vi "mod_truncate phase noise.vi"(0 "phase noise in":cluster{"f0":dbl, "df":dbl, "magnitude":dbl[]} {"f0" format="%.2p"; "df" format="%.2p"; "magnitude" format="%.2p"}, 5 "offset stop (Hz)":dbl=1000000.0 format="%.2p", 11 "error in (no error)":errorcluster) -> (4 "phase noise out (truncated)":cluster{"f0":dbl, "df":dbl, "magnitude":dbl[]} {"f0" format="%.2p"; "df" format="%.2p"; "magnitude" format="%.2p"}, 15 "error out":errorcluster)   [LabVIEW 2020, in "niAMT.lvlib"]
uses:
  <vilib>/addons/Modulation/niAMT.lvlib
panel:
  in  "offset stop (Hz)":dbl=900000.0 format="%.2p"
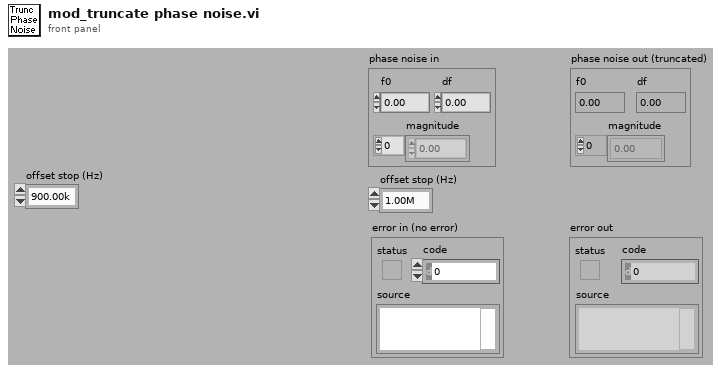
[diagram p1: front panel]
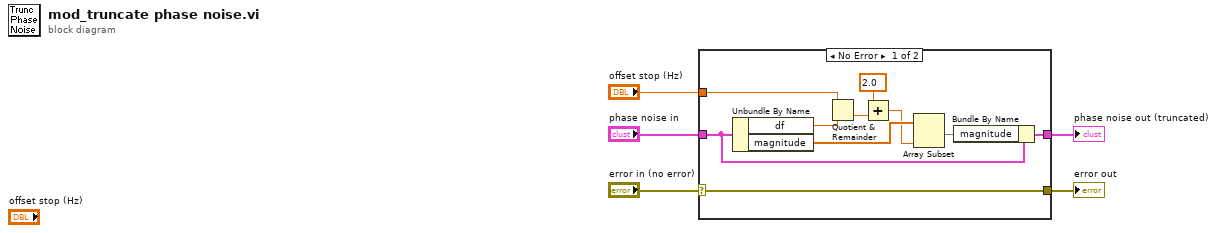
[diagram p0: block diagram]
diagram:
  n1 = case shown="No Error" "error in (no error)" {
    selector: "error in (no error)" -> [w6 w16]
    tunnel: "phase noise in" -> [w9 w17]
    tunnel: "offset stop (Hz)" -> [w8 _]
    tunnel: [w7 w17] -> w3
    tunnel: [w6 w16] -> w1
    frame No Error {
      n2 = Unbundle By Name(w9) -> ("df"=w15:dbl, "magnitude"=w14:dbl[])
      n3 = Quotient & Remainder(x=w8, y=w15) -> (floor(x/y)=w12:dbl)  [unwired: 1 out]
      n4 = Add(x=2.0, y=w12) -> (x+y=w10:dbl)
      n5 = Array Subset(array=w14, length=w10) -> (w13:dbl[])  [unwired: 1 in]
      n6 = Bundle By Name(cluster=w9, "magnitude"=w13) -> (w7:cluster{"f0":dbl, "df":dbl, "magnitude":dbl[]})
    }
    frame Error {
    }
  }
  "phase noise out (truncated)" <- w3
  "error out" <- w1
